vi "Master Setup Read Write File Errors.vi"(8 "error in (no error)":errorcluster, 9 "Read (F) Write (T)":bool, 10 "Pattern Label":T1 items=["Channel Setup (0)", "PID Setup (1)", "Filter Setup (2)", "~Reserved Old CAN Msgs (3)", "~Reserved Old CAN1 (4)", "~Reserved Old CAN2 (5)", "Digital Inputs Setup (6)", "Digital Outputs Setup (7)", "Logging 1 Setup (8)", "Logging 2 Setup (9)", "Logging 3 Setup (10)", "Setpoint Setup (11)", "Test Series Setup (12)", "Graph Setup (13)", "System Configure (14)", "Header (15)", "Profile Manager (16)", "Post-Mortem Logging (17)", "High-Speed Data (18)", "Statistic Channel Setup (19)", "Ramp Channel Setup (20)", "ETAS INCA Channel Setup (21)", "ETC ECCS Transducer Setup (22)", "ETC ECCS Test Setup (23)", "AVL AK Smoke Meter Setup (24)", "Triggers Setup (25)", "Alarm Limits Setup (26)", "YKWT1 Measurement (27)", "YKWT1 Instrument (28)", "Auto File Settings (29)", "Playback File Setting (30)", "UUT Constants (31)", "UPS Setup (32)", "Differential Channel Setup (33)", "Integral Channel Setup (34)", "Signal Channel Setup (35)", "Calibration Setup (36)", "BNC Setup (37)", "ASAP3 Setup (38)", "Chassis Force Calculations (39)", "Chassis Teststand Losses (40)", "Chassis Vehicle Losses (41)", "Formula Channels (42)", "ASAP3 Map Coords Setup (43)", "Digital Controls Setup (44)", "Push Buttons Setup (45)", "Sliders Setup (46)", "~Reserved~ (47)", "Email Setup (48)", "Timer Setup (49)", "Unit Conversion Setup (50)", "Visible Channels (51)", "Main Display Setup (52)", "Message Display Setup (53)", "Input Display Setup (54)", "Unico Parameter Downloads (55)", "Flow Meter Setup (56)", "Channel Zero Offset (57)", "YKWT2 Measurement (58)", "YKWT2 Instrument (59)", "~Reserved Old CAN3 (60)", "CAS Setup (61)", "Accumulation Channel Setup (62)", "Valvetrain Dynamics Setup (63)", "CCP Setup (64)", "System Log Setup (65)", "Throttle Controller (66)", "RE Shifter (67)", "Main Display (68)", "~Reserved~ (69)", "FlexRay (70)", "YKWT3 Measurement (71)", "YKWT3 Instrument (72)", "CAN XNET API (73)"], 11 "Reset":bool) -> (0 "error out":errorcluster, 3 "File Error (out)":bool[](array[boolean]))   [LabVIEW 2017]
uses:
  Master Setup Pattern Enum.ctl
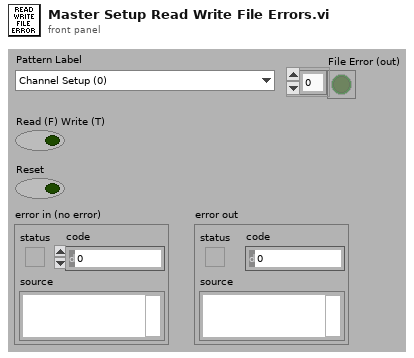
[diagram p1: front panel]
types:
  T1 = typedef "Master Setup Pattern Enum.ctl" = i32
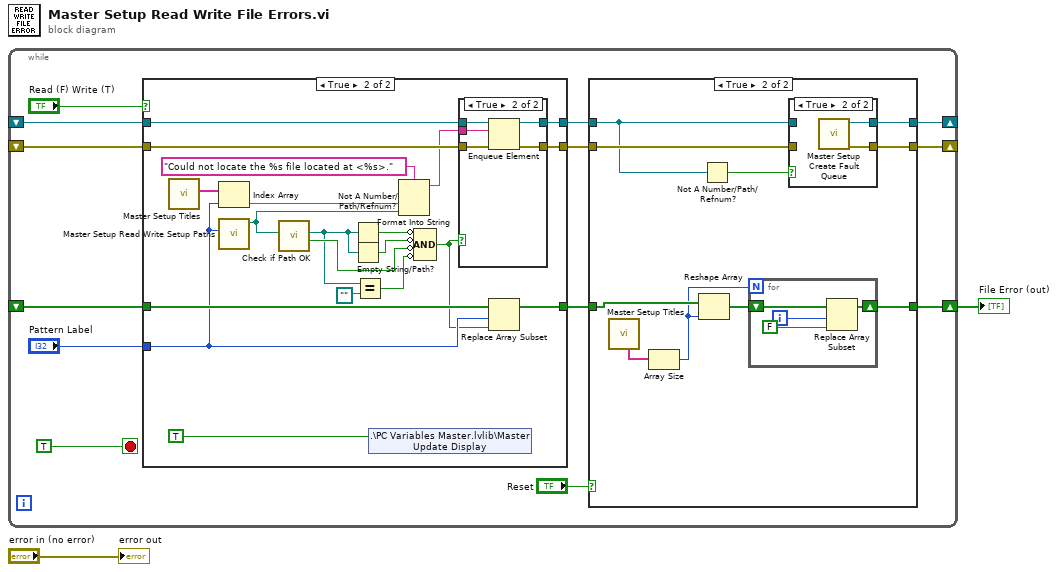
[diagram p0: block diagram]
diagram:
  n1 = while {
    shift-right: [w14] -> w2
    shift-left: _ -> [w13]
    shift-right: [w11] -> _
    shift-left: _ -> [w9]
    shift-right: [w10] -> _
    shift-left: _ -> [w7]
    stop <- TRUE stop-if-true
    n2 = case shown="True" "Read (F) Write (T)" {
      tunnel: [w18 w38] -> w12
      tunnel: w13 -> [w18 w37]
      tunnel: "Pattern Label" -> [_ w31]
      tunnel: w9 -> [w17 w35]
      tunnel: [w17 w34] -> w8
      tunnel: w7 -> [w16 w33]
      tunnel: [w16 w32] -> w6
      frame False {
      }
      frame True {
        n3 = call "Master Setup Titles.vi"() -> ("Setup Description"=w30:string[])  [unwired: 6 in, 5 out]
        n4 = Index Array(array=w30, index=w31) -> (element=w28:string)
        n5 = call "Master Setup Read Write Setup Paths.vi"("Pattern Label"=w31) -> ("New Setup Path"=w26:path)  [unwired: 6 in, 4 out]
        n6 = call "Check if Path OK.vi"("Path"=w26) -> ("Path OK"=w23:bool, "Path"=w20:path)  [unwired: 8 in, 1 out]
        n7 = Not A Number/Path/Refnum?(number/path/refnum=w20) -> (NaN/Path/Refnum?=w25:bool)
        n8 = Empty String/Path?(string/path=w20) -> (empty?=w24:bool)
        n9 = Equal?(x=w20, y=path "") -> (x = y?=w19:bool)
        n10 = shared-variable ".\\PC Variables Master.lvlib\\Master Update Display"(TRUE ("Master Update Display")) -> ()  [unwired: 1 in, 1 out]
        n11 = Format Into String(format string="Could not locate the %s file located at <%s>." ("[Date/Time] [Fault Status] [Fault Type] ... [Channel Name] ... [Value] ... [Limit]"), w28, w26) -> (resulting string=w27:string)  [unwired: 2 in, 1 out]
        n12 = Compound Arithmetic op=AND(invert w25, invert w24, invert w23, invert w19) -> (w22:bool)
        n13 = case shown="True" w22 {
          tunnel: w35 -> [w40 w45]
          tunnel: [w40 w44] -> w34
          tunnel: w33 -> [w39 w43]
          tunnel: [w39 w42] -> w32
          tunnel: w27 -> [_ w41]
          frame False {
          }
          frame True {
            n14 = Enqueue Element(queue=w45, element=w41, error in (no error)=w43) -> (queue out=w44:refnum<queue>, error out=w42:errorcluster)  [unwired: 1 in, 1 out]
          }
        }
        n15 = Replace Array Subset(array=w37, new element=w22, index=w31) -> (w38:bool[])
      }
    }
    n16 = case shown="True" "Reset" {
      tunnel: [w48 w50] -> w14
      tunnel: w12 -> [w48 w57]
      tunnel: [w47 w55] -> w11
      tunnel: w8 -> [w47 w52]
      tunnel: [w46 w54] -> w10
      tunnel: w6 -> [w46 w53]
      frame False {
      }
      frame True {
        n17 = call "Master Setup Titles.vi"() -> ("Sorted Setup Description"=w58:string[])  [unwired: 6 in, 5 out]
        n18 = Array Size(array=w58) -> (size(s)=w49:i32)
        n19 = Reshape Array(w57, w49) -> (w51:bool[])
        n20 = Not A Number/Path/Refnum?(number/path/refnum=w52) -> (NaN/Path/Refnum?=w56:bool)
        n21 = for {
          N: w49 -> [_]
          shift-right: [w61] -> w50
          shift-left: w51 -> [w62]
          i -> [w59]
          n22 = Replace Array Subset(array=w62, new element=FALSE ("new element/subarray"), index=w59) -> (w61:bool[])
        }
        n23 = case shown="True" w56 {
          tunnel: [w64 w66] -> w55
          tunnel: w52 -> [w64 _]
          tunnel: [w63 w65] -> w54
          tunnel: w53 -> [w63 _]
          frame False {
          }
          frame True {
            n24 = call "Master Setup Create Fault Queue.vi"() -> ("error out"=w65:errorcluster, "Master Fault Queue"=w66:refnum<queue>)  [unwired: 6 in]
          }
        }
      }
    }
  }
  "File Error (out)" <- w2
  "error out" <- "error in (no error)"
